vi "Initialize.vi"(0 "Program List in":refnum<class "Program List.lvclass">, 5 "error in (no error)":errorcluster, 8 "Application.lvclass":refnum<class "Application.lvclass">) -> (14 "Program List out":refnum<class "Program List.lvclass">, 19 "error out":errorcluster)   [LabVIEW 2019, in "Program List.lvclass"]
uses:
  Program List.lvclass
  Application.lvclass
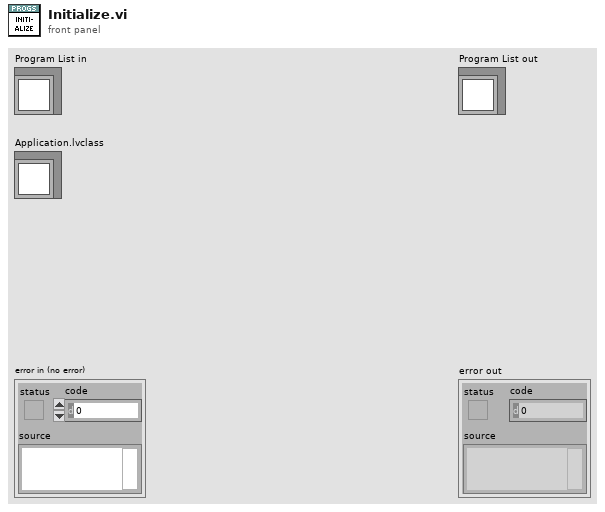
[diagram p1: front panel]
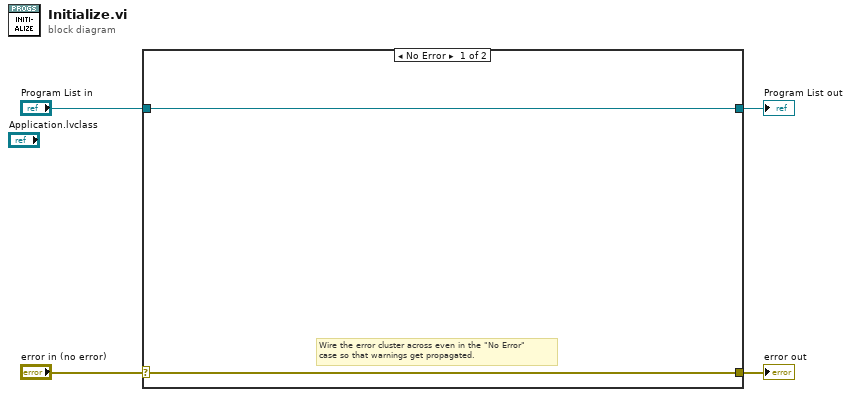
[diagram p0: block diagram]
diagram:
  n1 = case shown="No Error" "error in (no error)" {
    selector: "error in (no error)" -> [w5 w8]
    tunnel: [w5 w8] -> w3
    tunnel: [w6 w7] -> w1
    tunnel: "Program List in" -> [w6 w7]
    frame No Error {
      # "Wire the error cluster across even in the \"No Error\"\ncase so that warnings get propagated."
    }
    frame Error {
    }
  }
  "error out" <- w3
  "Program List out" <- w1
